vi "60 Get Joystick Input.vi"() -> ()   [LabVIEW 2018]
uses:
  <vilib>/Rock Robotics/WPI/Joystick/WPI_JoystickDeviceEnum.ctl
panel:
  out "POVs":i16[](array[numeric])
  out "Buttons":bool[](array[boolean])
  out "Axes":dbl[](array[numeric])
  in  "stop":bool
  out "Output":dbl(slide) scale=0.0..1.0
  out "Joystick X":dbl(slide) scale=1.0..-1.0
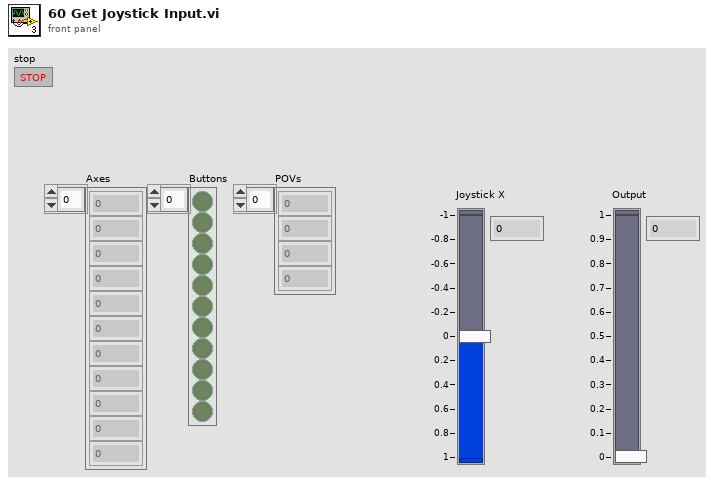
[diagram p1: front panel]
types:
  T1 = typedef "WPI_JoystickDeviceEnum.ctl" = enum16{"USB 0", "USB 1", "USB 2", "USB 3", "USB 4", "USB 5"}
  T2 = typedef "WPI_JoystickDevRef.ctl" = cluster{"Device":T1}
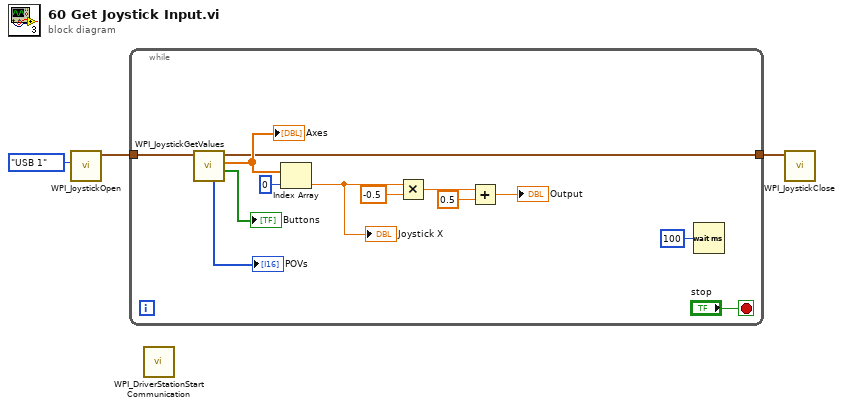
[diagram p0: block diagram]
diagram:
  n1 = call <vilib>:"WPI_JoystickOpen.vi"("JoystickDevice"=WPI_JoystickDeviceEnum."USB 1") -> ("JoystickDevRef"=w2:T2)  [unwired: 10 in]
  n2 = while {
    tunnel: w2 -> [w10]
    tunnel: [w6] -> w1
    stop <- "stop" stop-if-true
    n3 = call <vilib>:"WPI_JoystickGetValues.vi"("JoystickDevRef"=w10) -> ("Buttons"=→"Buttons":bool[], "Axes"=w9:dbl[], "JoystickDevRef"=w6:T2, "POVs"=→"POVs":i16[])  [unwired: 6 in, 1 out]
    "Axes" <- w9
    n4 = Index Array(array=w9, index=0) -> (element=w7:dbl)
    "Joystick X" <- w7
    n5 = Multiply(x=w7, y=-0.5) -> (x*y=w12:dbl)
    n6 = Add(x=w12, y=0.5) -> (x+y=→"Output":dbl)
    n7 = Wait (ms)(milliseconds to wait=u32 100) -> ()  [unwired: 1 out]
  }
  n8 = call <vilib>:"WPI_DriverStationStart Communication.vi"() -> ()  [unwired: 12 in]
  n9 = call <vilib>:"WPI_JoystickClose.vi"("JoystickDevRef"=w1) -> ()  [unwired: 11 in]
